vi "Main.vi"() -> ()   [LabVIEW 2017]
doc: "Top level UI for converting LabVIEW VIs into web format read by FINALE."
uses:
  PathConfiguration.vi
panel:
  in  "error in (no error)":errorcluster
  out "error out":errorcluster
  in  "Convert":bool
  in  "Destination Directory":path
  in  "Source directory/files":path
  out "Output":string
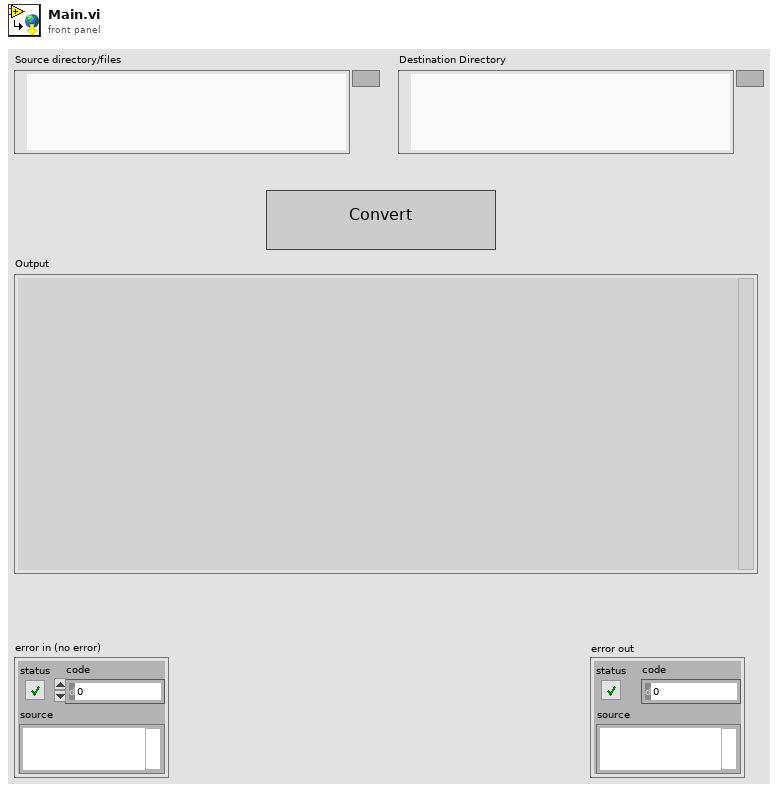
[diagram p1: front panel]
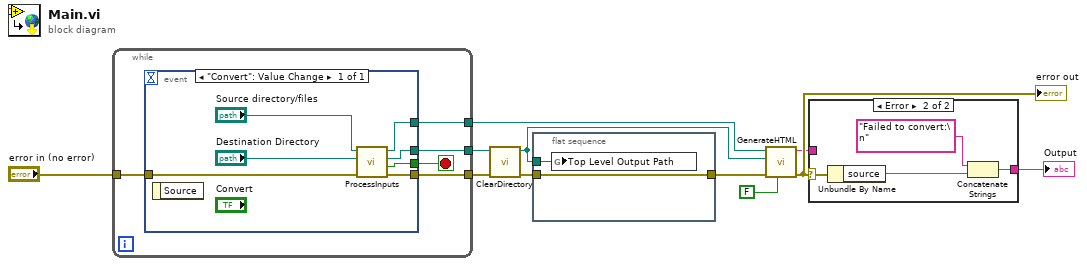
[diagram p0: block diagram]
diagram:
  n1 = while {
    tunnel: [w15] -> w6
    tunnel: [w14] -> w5
    tunnel: [w13] -> w11
    tunnel: "error in (no error)" -> [w12]
    stop <- w16 stop-if-true
    n2 = event shown="[0] \"Convert\": Value Change" {
      selector: _ -> [_]
      dyn-events: _ -> [_]
      timeout: _ -> [_]
      tunnel: [w19] -> w16
      tunnel: [w18] -> w15
      tunnel: [w20] -> w14
      tunnel: [w22] -> w13
      tunnel: w12 -> [w17]
      event "Convert": Value Change {
        n3 = event-data() -> ()  [unwired: 1 in, 1 out]
        n4 = call "ProcessInputs.vi"("error in (no error)"=w17, "Destination Directory"="Destination Directory", "Source directory/files"="Source directory/files") -> ("error out"=w18:errorcluster, "Continue?"=w19:bool, "Destination Directory out"=w20:path, "Source directory/files out"=w22:path)  [unwired: 5 in]
      }
    }
  }
  n5 = call "ClearDirectory.vi"("error in (no error)"=w6, "Directory in"=w5) -> ("error out"=w2:errorcluster, "Directory out"=w3:path)  [unwired: 8 in]
  n6 = flat-sequence {
    tunnel: w3 -> [w25]
    tunnel: w2 -> [w24]
    tunnel: [w24] -> w1
    frame #0 {
      n7 = global write "PathConfiguration.vi" "Top Level Output Path"(w25) -> ()
    }
  }
  n8 = call "GenerateHTML.vi"("Unattended Mode"=FALSE, "error in (no error)"=w1, "Destination Directory"=w3, "Source directory/files"=w11) -> ("error out"=w9:errorcluster, "Output"=w8:string)  [unwired: 6 in]
  "error out" <- w9
  n9 = case shown="Error" w9 {
    selector: w9 -> [_ w30]
    tunnel: w8 -> [w26 _]
    tunnel: [w26 w27] -> w7
    frame No Error {
    }
    frame Error {
      n10 = Unbundle By Name(w30) -> ("source"=w29:string)
      n11 = Concatenate Strings("Failed to convert:\n" ("string"), w29) -> (w27:string)
    }
  }
  "Output" <- w7
